vi "GetCaseDataType.vi"(6 "error in":errorcluster, 9 "CaseStructure in":refnum<class "CaseStructure.lvclass">) -> (0 "error out":errorcluster, 2 "Data Type":variant, 3 "CaseStructure out":refnum<class "CaseStructure.lvclass">)   [LabVIEW 2014, in "Raspberry Pi Compatible Compiler for LabVIEW.lvlib" / "CaseStructure.lvclass"]
uses:
  CaseStructure.lvclass
  Tunnel/Tunnel.lvclass
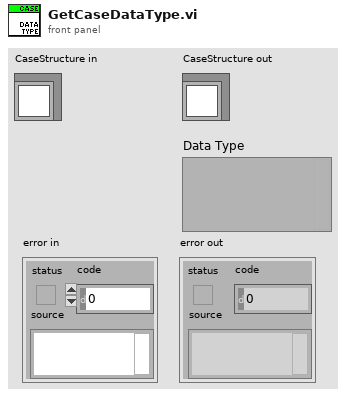
[diagram p1: front panel]
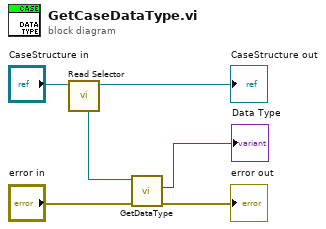
[diagram p0: block diagram]
diagram:
  n1 = call "Read Selector.vi"("CaseStructure in"="CaseStructure in") -> ("CaseStructure out"=→"CaseStructure out":refnum<class "CaseStructure.lvclass">, "Selector"=w4:refnum<class "Tunnel.lvclass">)  [unwired: 7 in]
  n2 = call "GetDataType.vi"("error in"="error in", "Tunnel in"=w4) -> ("error out"=→"error out":errorcluster, "Data Type"=→"Data Type":variant)  [unwired: 7 in, 1 out]
